vi "CLC_Gen4_L1_GUI_New.vi"() -> ()   [LabVIEW 2023, in "Clover_Cell.lvlib"]
uses:
  Clover_Cell.lvlib
panel:
  in  "Ch_4":i32
  in  "Ch_3":i32
  in  "Ch_2":i32
  in  "Ch_1":i32
  in  "Ch3_phase":i32=32 min=0 max=63 step=1
  in  "Ch2_phase":i32=32 min=0 max=63 step=1
  in  "Ch1_phase":i32 min=0 max=63 step=1
  in  "Ch4_phase":i32 min=0 max=63 step=1
  in  "Ch4_gain":i32 min=0 max=15 step=1
  in  "Ch3_gain":i32 min=0 max=15 step=1
  in  "Ch2_gain":i32 min=0 max=15 step=1
  in  "Ch1_gain":i32 min=0 max=15 step=1
  out "error out":errorcluster
  in  "Ethernet Setting":T1={"address"="192.168.100.111", "remote port or service name"=5025, "timeout ms (60000)"=10000}
  out "Status":bool
  in  "Ch2?":bool
  in  "Ch3?":bool
  in  "Ch4?":bool
  in  "Ch1?":bool
  in  "Polarity":u16(ring) items=["V", "H"]
  in  "TRXmode":u16(ring)=1 items=["Rx"=2, "Tx"=1]
  # "CLC_Gen4_L1 Setting GUI"
  # "Ch_On/OFF"
  # "Phase"
  # "Gain"
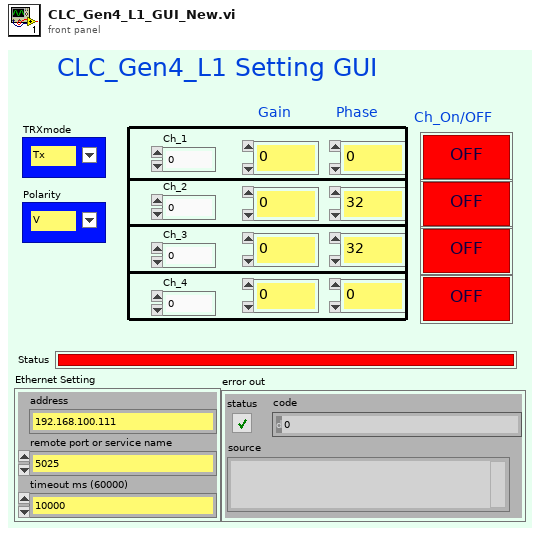
[diagram p1: front panel]
types:
  T1 = cluster{"address":string, "remote port or service name":u16, "timeout ms (60000)":i32}
  T2 = cluster{"Mode":u16, "Polarity":u16, "CH_ON/OFF":u16, "Channel":i32, "Gain":i32, "Phase":i32}
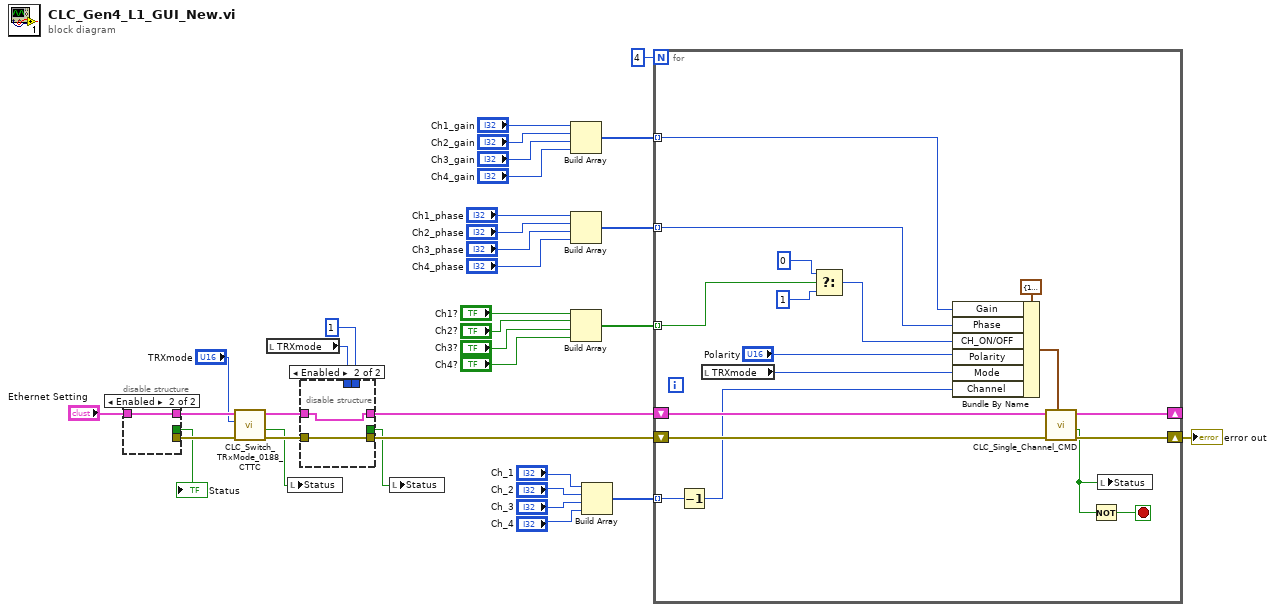
[diagram p0: block diagram]
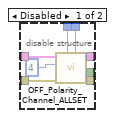
[diagram p2: hidden frame]
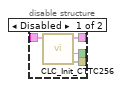
[diagram p3: hidden frame]
diagram:
  n1 = disable-structure shown="Enabled" {
    disable-tunnel: [w39 _] -> w35
    disable-tunnel: "Ethernet Setting" -> [w38 w40]
    disable-tunnel: [w37 w40] -> w32
    disable-tunnel: [w36 _] -> w13
    frame Disabled {
      n2 = call "CLC_Init_CTTC256.vi"("TCPIPin"=w38) -> ("error out"=w39:errorcluster, "Status"=w36:bool, "TCPIPin 2"=w37:T1)  [unwired: 8 in]
    }
    frame Enabled {
    }
  }
  "Status" <- w13
  n3 = call "CLC_Switch_TRxMode_0188_CTTC.vi"("error in (no error)"=w35, "Text Ring"="TRXmode", "TCPIPin"=w32) -> ("error out"=w34:errorcluster, "OK?"=w12:bool, "TCPIPin 2"=w30:T1)  [unwired: 6 in]
  n4 = local read "TRXmode"() -> (w29:u16)
  n5 = local write "Status"(w12) -> ()
  n6 = disable-structure shown="Enabled" {
    disable-tunnel: w34 -> [w48 w49]
    disable-tunnel: w30 -> [w46 w50]
    disable-tunnel: w29 -> [w45 _]
    disable-tunnel: u16 1 ("CH_ON:0/OFF:1") -> [w44 _]
    disable-tunnel: [w43 w49] -> w15
    disable-tunnel: [w42 w50] -> w14
    disable-tunnel: [w41 _] -> w11
    frame Disabled {
      n7 = call "OFF_Polarity_Channel_ALLSET.vi"("CH_ON:0/OFF:1"=w44, "Mode"=w45, "error in"=w48, "Channel"=4, "TCPIPin"=w46) -> ("error out"=w43:errorcluster, "OK?"=w41:bool, "TCPIPout"=w42:T1)  [unwired: 4 in]
    }
    frame Enabled {
    }
  }
  n8 = local write "Status"(w11) -> ()
  n9 = Build Array("Ch1_gain", "Ch2_gain", "Ch3_gain", "Ch4_gain") -> (w10:i32[])
  n10 = Build Array("Ch1_phase", "Ch2_phase", "Ch3_phase", "Ch4_phase") -> (w9:i32[])
  n11 = Build Array("Ch1?", "Ch2?", "Ch3?", "Ch4?") -> (w8:bool[])
  n12 = Build Array("Ch_1", "Ch_2", "Ch_3", "Ch_4") -> (w1:i32[])
  n13 = for {
    N: 4 -> [_]
    shift-right: [w64] -> w6
    shift-left: w15 -> [w65]
    shift-right: [w63] -> _
    shift-left: w14 -> [w66]
    tunnel: w10 -> [w62] mode=indexing
    tunnel: w9 -> [w61] mode=indexing
    tunnel: w8 -> [w58] mode=indexing
    tunnel: w1 -> [w52] mode=indexing
    stop <- w53 stop-if-true
    n14 = Decrement(x=w52) -> (x-1=w51:i32)
    n15 = local read "TRXmode"() -> (w60:u16)
    n16 = Select(t=u16 0 ("CH_ON/OFF"), s=w58, f=u16 1 ("CH_ON/OFF")) -> (s? t:f=w55:u16)
    n17 = Bundle By Name(cluster=T2 {"Mode"=1, "Polarity"=1, "CH_ON/OFF"=1, "Channel"=0, "Gain"=0, "Phase"=0} ("Channel params"), "Gain"=w62, "Phase"=w61, "CH_ON/OFF"=w55, "Polarity"="Polarity", "Mode"=w60, "Channel"=w51) -> (w67:T2)
    n18 = call "CLC_Single_Channel_CMD.vi"("Channel params"=w67, "error in"=w65, "TCPIPin"=w66) -> ("error out"=w64:errorcluster, "OK?"=w54:bool, "TCPIPout"=w63:T1)  [unwired: 6 in]
    n19 = Not(x=w54) -> (.not. x?=w53:bool)
    n20 = local write "Status"(w54) -> ()
  }
  "error out" <- w6
